vi "CopyAllData2D.vi"(8 "error in (no error)":errorcluster) -> (0 "error out":errorcluster, 1 "data1":u16[][](array[numeric]), 2 "data0":u16[][](array[numeric]))   [LabVIEW 2015, in "ESLSCDLL.lvlib"]
uses:
  ESLSCDLL.lvlib
  Globals.vi
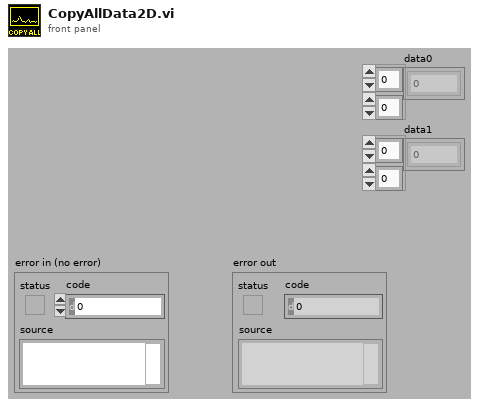
[diagram p1: front panel]
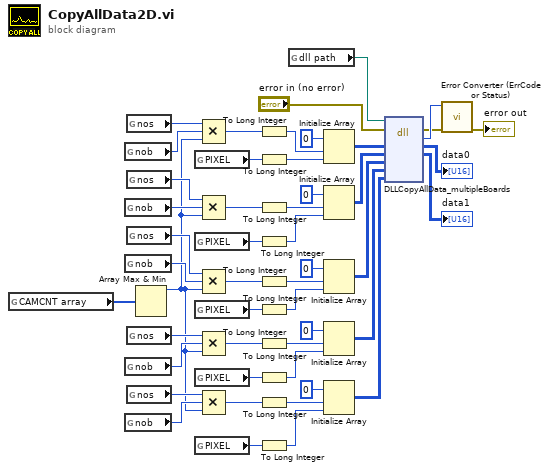
[diagram p0: block diagram]
diagram:
  n1 = global read "Globals.vi" "CAMCNT array"() -> (w36:u32[])
  n2 = global read "Globals.vi" "nob"() -> (w45:u32)
  n3 = global read "Globals.vi" "nob"() -> (w39:u32)
  n4 = global read "Globals.vi" "nob"() -> (w32:u32)
  n5 = global read "Globals.vi" "nob"() -> (w27:u32)
  n6 = global read "Globals.vi" "nob"() -> (w22:u32)
  n7 = global read "Globals.vi" "nos"() -> (w44:u32)
  n8 = global read "Globals.vi" "nos"() -> (w38:u32)
  n9 = global read "Globals.vi" "nos"() -> (w31:u32)
  n10 = global read "Globals.vi" "nos"() -> (w26:u32)
  n11 = global read "Globals.vi" "nos"() -> (w21:u32)
  n12 = Array Max & Min(array=w36) -> (max value=w20:u32)  [unwired: 3 out]
  n13 = global read "Globals.vi" "PIXEL"() -> (w16:u32)
  n14 = global read "Globals.vi" "PIXEL"() -> (w14:u32)
  n15 = global read "Globals.vi" "PIXEL"() -> (w12:u32)
  n16 = global read "Globals.vi" "PIXEL"() -> (w10:u32)
  n17 = global read "Globals.vi" "PIXEL"() -> (w8:u32)
  n18 = Compound Arithmetic op=MULTIPLY(w44, w45, w20) -> (w46:u32)
  n19 = Compound Arithmetic op=MULTIPLY(w38, w39, w20) -> (w40:u32)
  n20 = Compound Arithmetic op=MULTIPLY(w31, w32, w20) -> (w33:u32)
  n21 = Compound Arithmetic op=MULTIPLY(w26, w27, w20) -> (w28:u32)
  n22 = Compound Arithmetic op=MULTIPLY(w21, w22, w20) -> (w23:u32)
  n23 = To Long Integer(number=w46) -> (32bit integer=w48:i32)
  n24 = To Long Integer(number=w16) -> (32bit integer=w15:i32)
  n25 = To Long Integer(number=w40) -> (32bit integer=w42:i32)
  n26 = To Long Integer(number=w14) -> (32bit integer=w13:i32)
  n27 = To Long Integer(number=w33) -> (32bit integer=w35:i32)
  n28 = To Long Integer(number=w12) -> (32bit integer=w11:i32)
  n29 = To Long Integer(number=w28) -> (32bit integer=w30:i32)
  n30 = To Long Integer(number=w10) -> (32bit integer=w9:i32)
  n31 = To Long Integer(number=w23) -> (32bit integer=w25:i32)
  n32 = To Long Integer(number=w8) -> (32bit integer=w7:i32)
  n33 = global read "Globals.vi" "dll path"() -> (w1:path)
  n34 = Initialize Array(u16 0, w48, w15) -> (w43:u16[][])
  n35 = Initialize Array(u16 0, w42, w13) -> (w37:u16[][])
  n36 = Initialize Array(u16 0, w35, w11) -> (w19:u16[][])
  n37 = Initialize Array(u16 0, w30, w9) -> (w18:u16[][])
  n38 = Initialize Array(u16 0, w25, w7) -> (w17:u16[][])
  n39 = dll-call lib="C:/ENTW/PCIE/LV64/board.vis/ESLSCDLL.dll" fn="DLLCopyAllData_multipleBoards" ("lwlscdll.dll:DLLReadLongS0")(path in=w1, error in="error in (no error)", "pdest0"=w43, "pdest1"=w37, "pdest2"=w19, "pdest3"=w18, "pdest4"=w17) -> (error out=w3:errorcluster, "es_status_codes"=w4:i32, "pdest0"=→"data0":u16[][], "pdest1"=→"data1":u16[][])  [unwired: 4 in, 1 out]
  n40 = call "Error Converter (ErrCode or Status).vi"("error in (no error)"=w3, "error code"=w4) -> ("error out"=→"error out":errorcluster)  [unwired: 9 in]
